vi "读取数据文件.vi"(8 "错误输入（无错误）":errorcluster, 11 "tdms文件路径":path) -> (0 "错误输出":errorcluster, 3 "数据":T1)   [LabVIEW 2021]
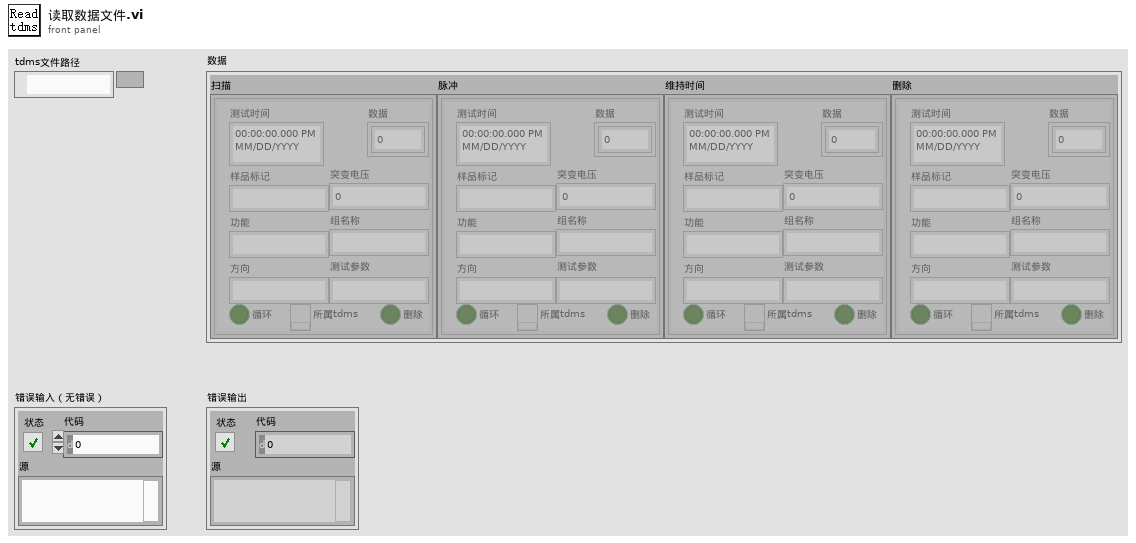
[diagram p1: front panel]
types:
  T1 = typedef "缓冲数据.ctl" = cluster{"扫描":T2[], "脉冲":T2[], "维持时间":T2[], "删除":T2[]}
  T2 = typedef "测试数据类型.ctl" = cluster{"测试时间":timestamp, "数据":dbl[][], "功能":string, "方向":string, "循环":bool, "样品标记":string, "突变电压":i32, "所属tdms":refnum<k34>, "组名称":string, "删除":bool, "测试参数":string}
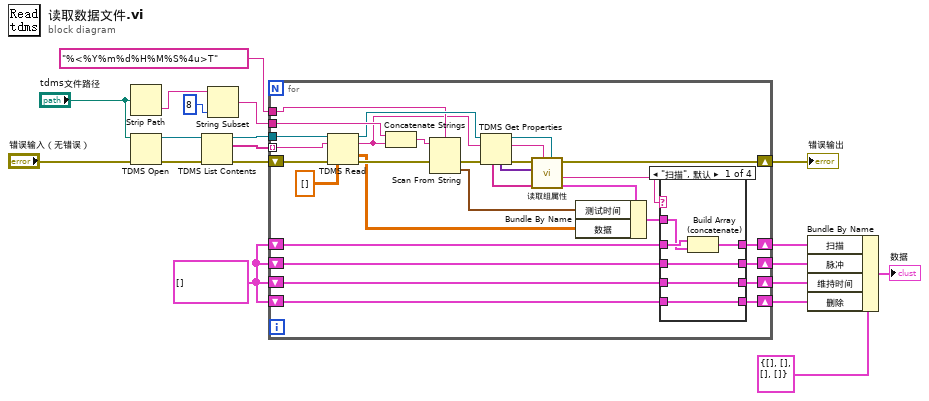
[diagram p0: block diagram]
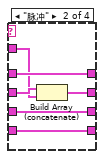
[diagram p2: hidden frame]
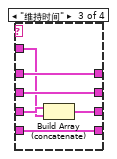
[diagram p3: hidden frame]
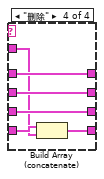
[diagram p4: hidden frame]
diagram:
  w3 = T2[] []
  n1 = Strip Path(path="tdms文件路径") -> (name=w15:string)  [unwired: 1 out]
  n2 = TDMS Open(8:"错误输入（无错误）", 11:"tdms文件路径") -> (0:w11:errorcluster, 3:w19:refnum<k34>)  [unwired: 5 in]
  n3 = TDMS List Contents(4:w11, 7:w19) -> (0:w12:errorcluster, 2:w17:string[], 3:w18:refnum<k34>)  [unwired: 1 in, 1 out]
  n4 = String Subset(string=w15, length (rest)=8 ("长度（剩余）")) -> (substring=w13:string)  [unwired: 1 in]
  n5 = for {
    tunnel: w18 -> [w49]
    tunnel: w17 -> [w38] mode=indexing
    tunnel: w13 -> [w47]
    shift-right: [w44] -> w6
    shift-left: w3 -> [w43]
    shift-right: [w42] -> w5
    shift-left: w3 -> [w41]
    shift-right: [w40] -> w4
    shift-left: w3 -> [w39]
    shift-right: [w33] -> w9
    shift-left: w12 -> [w27]
    shift-right: [w36] -> w2
    shift-left: w3 -> [w37]
    tunnel: "%<%Y%m%d%H%M%S%4u>T" ("格式字符串") -> [w22]
    n6 = TDMS Read(0:w49, 5:w38, 11:w27, 12:dbl[][] []) -> (4:w46:refnum<k34>, 6:w20:string, 10:w21:dbl[][], 15:w24:errorcluster)  [unwired: 4 in, 2 out]
    n7 = Concatenate Strings(w47, w20) -> (w45:string)
    n8 = Scan From String(format string=w22, input string=w45, error in=w24) -> (error out=w23:errorcluster, output 1=w30:timestamp)  [unwired: 2 in, 2 out]
    n9 = TDMS Get Properties(8:w23, 10:w20, 11:w46) -> (0:w34:errorcluster, 2:w26:string, 3:w25:refnum<k34>, 4:w29:variant[], 6:w32:string[])  [unwired: 3 in, 1 out]
    n10 = call "读取组属性.vi"("tdms文件输出"=w25, "组名称"=w26, "属性名称"=w32, "属性值"=w29, "错误输入（无错误）"=w34) -> ("测试数据"=w31:T2, "数据类型"=w28:string, "错误输出"=w33:errorcluster)  [unwired: 4 in]
    n11 = Bundle By Name(cluster=w31, "测试时间"=w30, "数据"=w21) -> (w35:T2)
    n12 = case shown="\"扫描\", 默认" w28 {
      tunnel: [w55 w58 w64 w71] -> w44
      tunnel: w43 -> [w54 w58 w64 w71]
      tunnel: [w52 w61 w63 w70] -> w42
      tunnel: w41 -> [w52 w60 w63 w70]
      tunnel: [w51 w57 w67 w69] -> w40
      tunnel: w39 -> [w51 w57 w66 w69]
      tunnel: w35 -> [w50 w56 w62 w68]
      tunnel: w37 -> [w53 w59 w65 w73]
      tunnel: [w53 w59 w65 w72] -> w36
      frame "扫描", Default {
        n13 = Build Array (concatenate)(w54, w50) -> (w55:T2[])
      }
      frame "脉冲" {
        n14 = Build Array (concatenate)(w60, w56) -> (w61:T2[])
      }
      frame "维持时间" {
        n15 = Build Array (concatenate)(w66, w62) -> (w67:T2[])
      }
      frame "删除" {
        n16 = Build Array (concatenate)(w73, w68) -> (w72:T2[])
      }
    }
  }
  "错误输出" <- w9
  n17 = Bundle By Name(cluster=T1 {"扫描"=[], "脉冲"=[], "维持时间"=[], "删除"=[]} ("数据"), "扫描"=w6, "脉冲"=w5, "维持时间"=w4, "删除"=w2) -> (→"数据":T1)
